vi "Explorer_List.vi"() -> (1 "Options":string[](array[string]), 2 "Explore Path":path, 3 "Files":path[](array[path]))   [LabVIEW 2022 SP3]
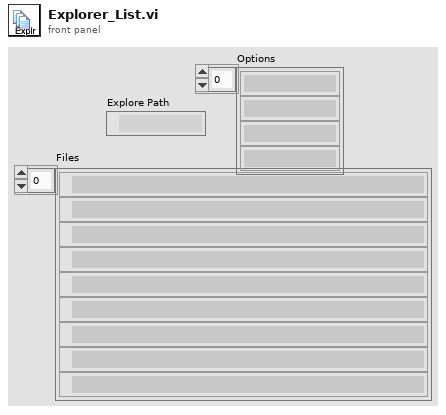
[diagram p1: front panel]
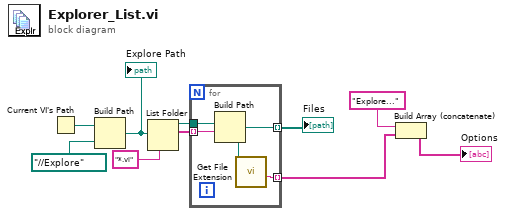
[diagram p0: block diagram]
diagram:
  n1 = Current VI's Path() -> (path=w5:path)
  n2 = Build Path(base path=w5, name or relative path=path "../../Explore") -> (appended path=w10:path)
  "Explore Path" <- w10
  n3 = List Folder(path=w10, pattern="*.vi") -> (path out=w9:path, filenames=w8:string[])  [unwired: 2 in, 2 out]
  n4 = for {
    tunnel: w9 -> [w14]
    tunnel: w8 -> [w13] mode=indexing
    tunnel: [w12] -> w7 mode=indexing
    tunnel: [w11] -> w2 mode=indexing
    n5 = Build Path(base path=w14, name or relative path=w13) -> (appended path=w12:path)
    n6 = call <vilib>:"Get File Extension.vi"("file"=w12) -> ("filename without extension"=w11:string)  [unwired: 6 in, 4 out]
  }
  "Files" <- w7
  n7 = Build Array (concatenate)("Explore...", w2) -> (→"Options":string[])
